vi "批量读D+10个+16位.vi"(8 "error out":errorcluster, 10 "读取D地址":i32, 11 "VISA resource name out":refnum<visa-resource-name>) -> (0 "error IO":errorcluster, 1 "读取缓冲区":string, 2 "数组":i32[](array[numeric]), 3 "VISA resource name out 2":refnum<visa-resource-name>)   [LabVIEW 2018]
uses:
  <vilib>/Instr/_visa.llb/VISA Configure Serial Port (Instr).vi
panel:
  out "连接的字符串 2":string
  out "连接的字符串":string
  out "通讯延时":u32
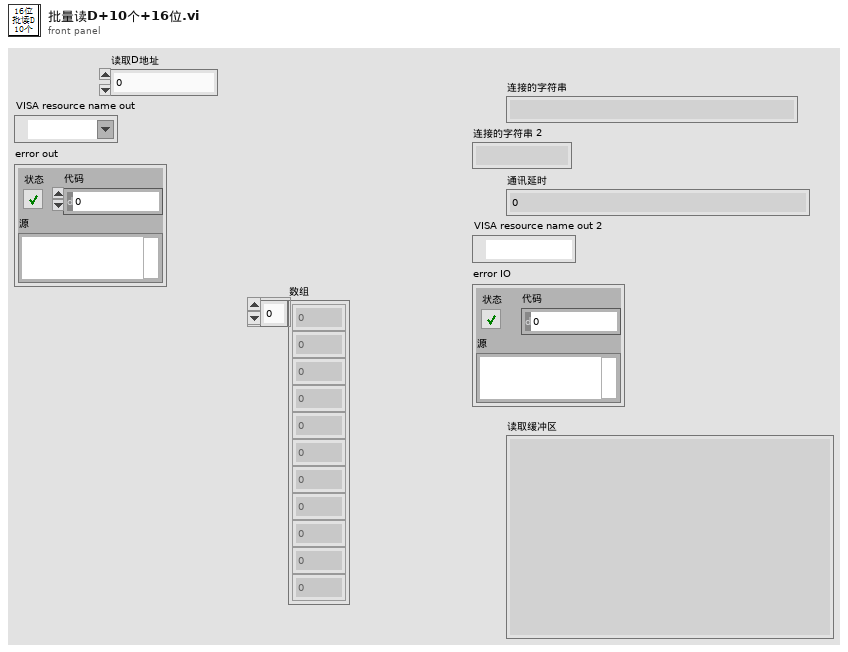
[diagram p1: front panel]
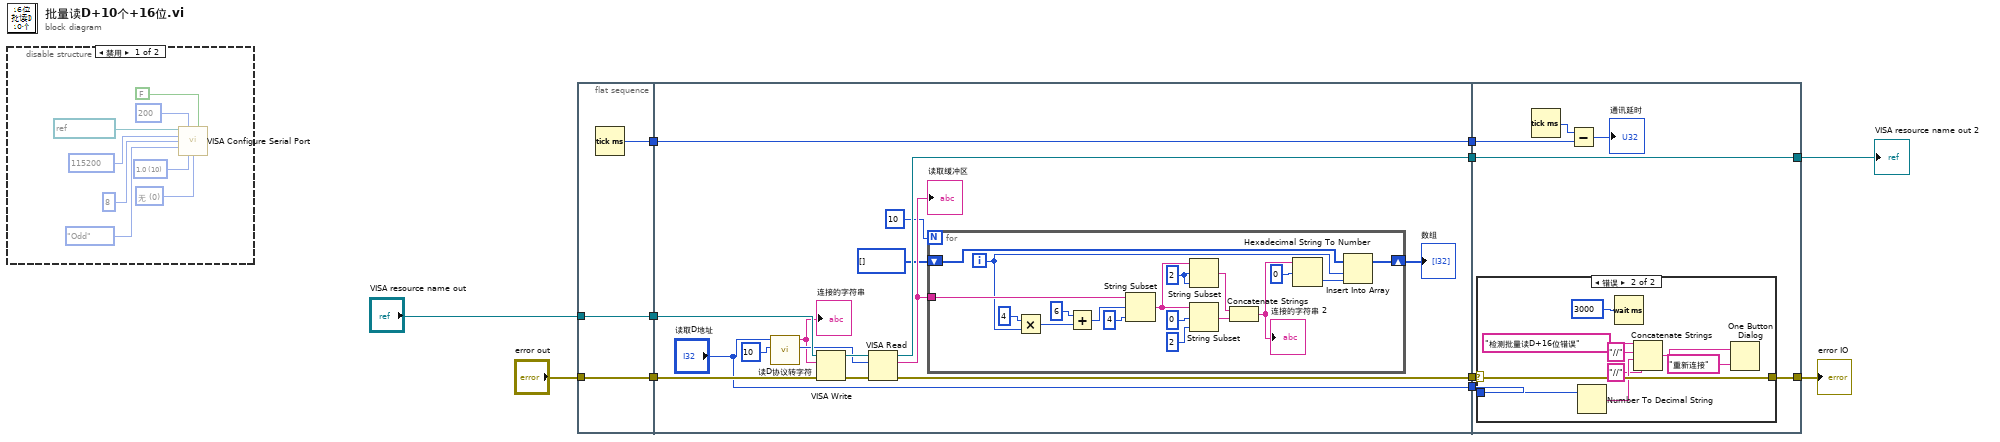
[diagram p0: block diagram]
diagram:
  n1 = disable-structure shown="禁用" {
    frame Disabled {
      w13 = u16 0 items=["无", "XON/XOFF", "RTS/CTS", "XON/XOFF & RTS/CTS", "DTR/DSR", "XON/XOFF & DTR/DSR"] ("flow control (0:none)")
      w14 = u16 10 items=["1.0"=10, "1.5"=15, "2.0"=20] ("stop bits (10: 1 bit)")
      n2 = call-poly "VISA Configure Serial Port"("VISA resource name"=refnum<visa-resource-name> "COM3", "timeout (10sec)"=u32 200, "Enable Termination\nChar (T)"=FALSE ("Enable Termination\nChar (T)"), "baud rate (9600)"=u32 115200, "data bits (8)"=u16 8, "parity (0:none)"=enum16{"None", "Odd", "Even", "Mark", "Space"}."Odd", "stop bits (10: 1 bit)"=w14, "flow control (0:none)"=w13) -> ()  [unwired: 6 in, 2 out]
    }
    frame Enabled {
    }
  }
  n3 = flat-sequence {
    tunnel: [w22] -> w11
    tunnel: "VISA resource name out" -> [w21]
    tunnel: [w21] -> w10
    tunnel: [w20] -> w9
    tunnel: "error out" -> [w20]
    tunnel: w11 -> [w37]
    tunnel: [w37] -> w8
    tunnel: [w36] -> w7
    tunnel: [w35] -> w6
    tunnel: w10 -> [w34]
    tunnel: w9 -> [w33]
    tunnel: ["读取D地址"] -> w1
    tunnel: w8 -> [w61]
    tunnel: w7 -> [w59]
    tunnel: [w59] -> w3
    tunnel: w6 -> [w58]
    tunnel: [w57] -> w2
    tunnel: w1 -> [w56]
    frame #0 {
      n4 = Tick Count (ms)() -> (millisecond timer value=w22:u32)
    }
    frame #1 {
      n5 = call "读D协议转字符.vi"("读取D个数"=10, "读取D地址"="读取D地址") -> ("读取的字节数"=w30:i32, "连接的字符串"=w29:string)  [unwired: 8 in]
      "连接的字符串" <- w29
      n6 = VISA Write(VISA resource name=w34, write buffer=w29, error in (no error)=w33) -> (VISA resource name out=w32:refnum<visa-resource-name>, error out=w31:errorcluster)  [unwired: 1 out]
      n7 = VISA Read(VISA resource name=w32, byte count=w30, error in (no error)=w31) -> (VISA resource name out=w36:refnum<visa-resource-name>, read buffer=w28:string, error out=w35:errorcluster)  [unwired: 1 out]
      "读取缓冲区" <- w28
      n8 = for {
        N: 10 -> [_]
        tunnel: w28 -> [w55]
        shift-right: [w53] -> w24
        shift-left: i32[] [] -> [w54]
        i -> [w51]
        w44 = 2 ("偏移量(0)")
        n9 = Multiply(x=4, y=w51) -> (x*y=w48:i32)
        n10 = Add(x=6 ("偏移量(0)"), y=w48) -> (x+y=w47:i32)
        n11 = String Subset(string=w55, offset (0)=w47, length (rest)=4 ("长度（剩余）")) -> (substring=w39:string)
        n12 = String Subset(string=w39, offset (0)=w44, length (rest)=w44) -> (substring=w42:string)
        n13 = String Subset(string=w39, offset (0)=0 ("偏移量(0)"), length (rest)=2 ("长度（剩余）")) -> (substring=w43:string)
        n14 = Concatenate Strings(w42, w43) -> (w41:string)
        "连接的字符串 2" <- w41
        n15 = Hexadecimal String To Number(string=w41, offset=0 ("偏移量")) -> (number=w38:u32)  [unwired: 1 in, 1 out]
        n16 = Insert Into Array(array=w54, index=w51, new element=w38) -> (w53:i32[])
      }
      "数组" <- w24
    }
    frame #2 {
      n17 = case shown="错误" w58 {
        selector: w58 -> [w63 w72]
        tunnel: [w63 w72] -> w57
        tunnel: w56 -> [_ w69]
        frame No Error {
        }
        frame Error {
          n18 = Number To Decimal String(number=w69) -> (decimal integer string=w66:string)  [unwired: 1 in]
          n19 = Wait (ms)(milliseconds to wait=u32 3000 ("等待时间（毫秒）")) -> ()  [unwired: 1 out]
          n20 = Concatenate Strings("检测批量读D+16位错误" ("消息"), "//" ("字符串"), w66, "//" ("字符串")) -> (w64:string)
          n21 = One Button Dialog(message=w64, button name ("OK")="重新连接" ("按钮名称（“确定”）")) -> ()  [unwired: 1 out]
        }
      }
      n22 = Tick Count (ms)() -> (millisecond timer value=w62:u32)
      n23 = Subtract(x=w62, y=w61) -> (x-y=→"通讯延时":u32)
    }
  }
  "VISA resource name out 2" <- w3
  "error IO" <- w2
